vi "main2.vi"() -> ()   [LabVIEW 2012]
uses:
  Global1.vi
panel:
  out "String":string
  out "Lot":string
  in  "folder":string="QAMT01\\CRH3605"
  out "f":bool
  out "after substring":string
  out "before substring":string
  out "text":string
  out "error out":errorcluster
  in  "error in (no error)":errorcluster
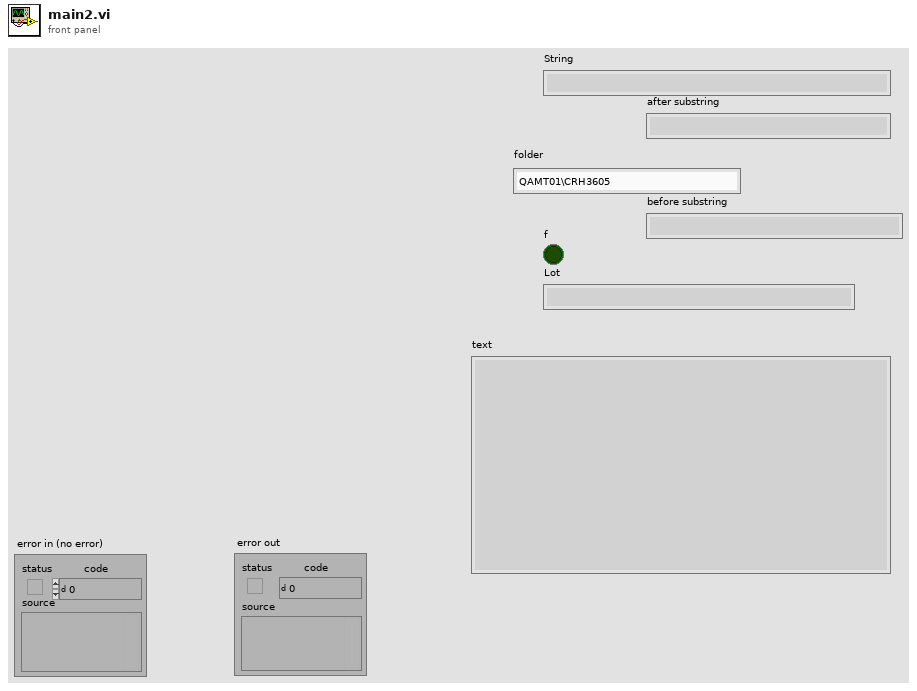
[diagram p1: front panel]
types:
  T1 = enum16{"open", "replace", "create", "open or create", "replace or create", "replace or create with confirmation"}
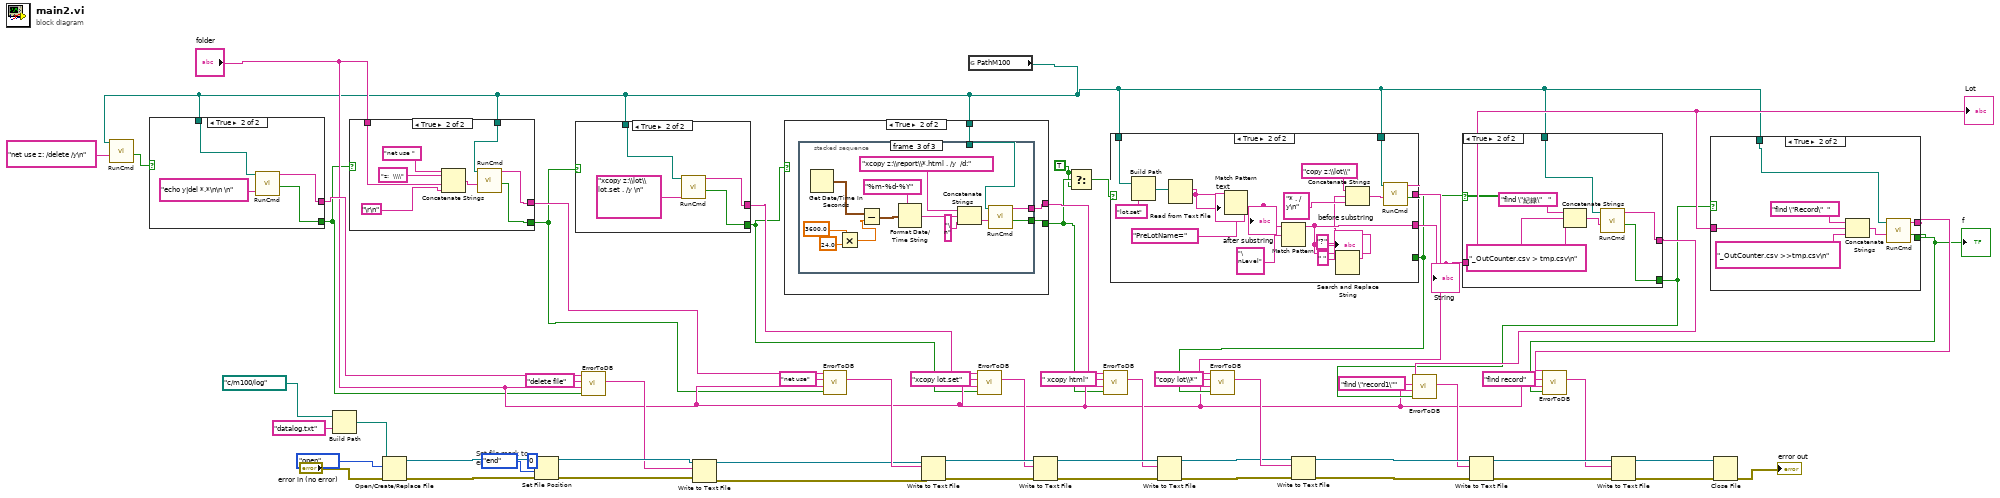
[diagram p0: block diagram]
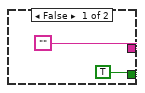
[diagram p2: hidden frame]
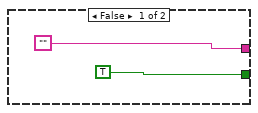
[diagram p3: hidden frame]
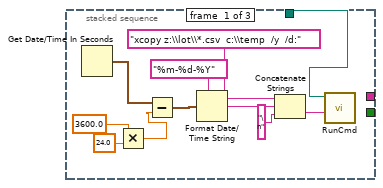
[diagram p4: hidden frame]
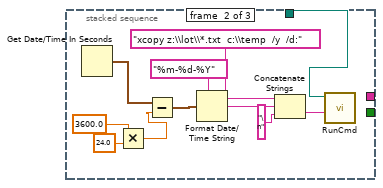
[diagram p5: hidden frame]
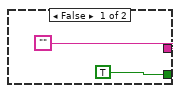
[diagram p6: hidden frame]
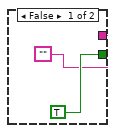
[diagram p7: hidden frame]
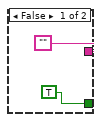
[diagram p8: hidden frame]
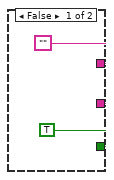
[diagram p9: hidden frame]
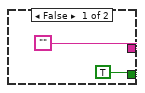
[diagram p10: hidden frame]
diagram:
  w6 = TRUE
  # "Set file mark to\nend of file"
  n1 = Build Path(base path=path "c:/m100/log", name or relative path="datalog.txt") -> (appended path=w53:path)
  n2 = Open/Create/Replace File(file path (use dialog)=w53, error in="error in (no error)", operation (0:open)=T1."open") -> (refnum out=w58:refnum<file>, error out=w57:errorcluster)  [unwired: 3 in, 1 out]
  n3 = Set File Position(offset (in bytes) (0)=i64 0, refnum=w58, from (0:start)=enum16{"start", "end", "current"}."end", error in=w57) -> (refnum out=w22:refnum<file>, error out=w21:errorcluster)
  n4 = global read "Global1.vi" "PathM100"() -> (w5:path)
  n5 = call "RunCmd.vi"("Cmd String"="net use z: /delete /y\n" ("string"), "working directory"=w5) -> ("OK"=w23:bool)  [unwired: 8 in, 1 out]
  n6 = case shown="True" w23 {
    tunnel: [TRUE w65] -> w3
    tunnel: ["" w64] -> w18
    tunnel: w5 -> [_ w67]
    frame False {
    }
    frame True {
      n7 = call "RunCmd.vi"("Cmd String"="echo y|del *.*\n\n \n" ("standard input"), "working directory"=w67) -> ("OK"=w65:bool, "Output"=w64:string)  [unwired: 8 in]
    }
  }
  n8 = case shown="True" w3 {
    tunnel: [TRUE w70] -> w4
    tunnel: ["" w71] -> w31
    tunnel: "folder" -> [_ w73]
    tunnel: w5 -> [_ w72]
    frame False {
    }
    frame True {
      n9 = Concatenate Strings("net use " ("string"), "z:  \\\\" ("string"), w73, "\r\n") -> (w77:string)
      n10 = call "RunCmd.vi"("Cmd String"=w77, "working directory"=w72) -> ("OK"=w70:bool, "Output"=w71:string)  [unwired: 8 in]
    }
  }
  n11 = case shown="True" w4 {
    tunnel: [TRUE w81] -> w2
    tunnel: ["" w80] -> w30
    tunnel: w5 -> [_ w83]
    frame False {
    }
    frame True {
      n12 = call "RunCmd.vi"("Cmd String"="xcopy z:\\lot\\lot.set . /y \n" ("standard input"), "working directory"=w83) -> ("OK"=w81:bool, "Output"=w80:string)  [unwired: 8 in]
    }
  }
  n13 = call "ErrorToDB.vi"("Error"=w3, "Folder"="folder", "Command"="delete file", "Error Message"=w18) -> ("LogData"=w17:string)  [unwired: 7 in]
  n14 = Write to Text File(file (use dialog)=w22, text=w17, error in=w21) -> (refnum out=w20:refnum<file>, error out=w19:errorcluster)  [unwired: 1 in, 1 out]
  n15 = case shown="True" w2 {
    tunnel: [TRUE w86] -> w8
    tunnel: ["" w87] -> w29
    tunnel: w5 -> [_ w88]
    frame False {
    }
    frame True {
      n16 = stacked-sequence {
        tunnel: w88 -> [w89 w100 w113]
        tunnel: [_ _ w112] -> w87
        tunnel: [_ _ w111] -> w86
        frame #0 {
          n17 = Get Date/Time In Seconds() -> (seconds since 1Jan1904=w90:timestamp)
          n18 = Multiply(x=3600.0, y=24.0) -> (x*y=w92:dbl)
          n19 = Subtract(x=w90, y=w92) -> (x-y=w93:timestamp)
          n20 = Format Date/Time String(time format string (%c)="%m-%d-%Y", seconds (now)=w93) -> (date/time string=w96:string)  [unwired: 1 in]
          n21 = Concatenate Strings("xcopy z:\\lot\\*.csv  c:\\temp  /y  /d:" ("string"), w96, "\n" ("string")) -> (w99:string)
          n22 = call "RunCmd.vi"("Cmd String"=w99, "working directory"=w89) -> ()  [unwired: 8 in, 2 out]
        }
        frame #1 {
          n23 = Get Date/Time In Seconds() -> (seconds since 1Jan1904=w101:timestamp)
          n24 = Multiply(x=3600.0, y=24.0) -> (x*y=w103:dbl)
          n25 = Subtract(x=w101, y=w103) -> (x-y=w104:timestamp)
          n26 = Format Date/Time String(time format string (%c)="%m-%d-%Y", seconds (now)=w104) -> (date/time string=w107:string)  [unwired: 1 in]
          n27 = Concatenate Strings("xcopy z:\\lot\\*.txt  c:\\temp  /y  /d:" ("string"), w107, "\n" ("string")) -> (w110:string)
          n28 = call "RunCmd.vi"("Cmd String"=w110, "working directory"=w100) -> ()  [unwired: 8 in, 2 out]
        }
        frame #2 {
          n29 = Get Date/Time In Seconds() -> (seconds since 1Jan1904=w114:timestamp)
          n30 = Multiply(x=3600.0, y=24.0) -> (x*y=w116:dbl)
          n31 = Subtract(x=w114, y=w116) -> (x-y=w117:timestamp)
          n32 = Format Date/Time String(time format string (%c)="%m-%d-%Y", seconds (now)=w117) -> (date/time string=w120:string)  [unwired: 1 in]
          n33 = Concatenate Strings("xcopy z:\\report\\*.html . /y  /d:" ("string"), w120, "\n" ("string")) -> (w123:string)
          n34 = call "RunCmd.vi"("Cmd String"=w123, "working directory"=w113) -> ("OK"=w111:bool, "Output"=w112:string)  [unwired: 8 in]
        }
      }
    }
  }
  n35 = call "ErrorToDB.vi"("Error"=w4, "Folder"="folder", "Command"="net use", "Error Message"=w31) -> ("LogData"=w43:string)  [unwired: 7 in]
  n36 = Write to Text File(file (use dialog)=w20, text=w43, error in=w19) -> (refnum out=w52:refnum<file>, error out=w51:errorcluster)  [unwired: 1 in, 1 out]
  n37 = call "ErrorToDB.vi"("Error"=w2, "Folder"="folder", "Command"="xcopy lot.set", "Error Message"=w30) -> ("LogData"=w42:string)  [unwired: 7 in]
  n38 = Write to Text File(file (use dialog)=w52, text=w42, error in=w51) -> (refnum out=w28:refnum<file>, error out=w27:errorcluster)  [unwired: 1 in, 1 out]
  n39 = Select(t=w6, s=w8, f=w6) -> (s? t:f=w7:bool)
  n40 = call "ErrorToDB.vi"("Error"=w8, "Folder"="folder", "Command"=" xcopy html", "Error Message"=w29) -> ("LogData"=w24:string)  [unwired: 7 in]
  n41 = case shown="True" w7 {
    tunnel: [TRUE w130] -> w38
    tunnel: [w124 w131] -> w39
    tunnel: w5 -> [_ w134]
    tunnel: [w124 w127] -> w44
    tunnel: w5 -> [_ w132]
    frame False {
      w124 = ""
    }
    frame True {
      n42 = Build Path(base path=w134, name or relative path="lot.set") -> (appended path=w142:path)
      n43 = Read from Text File(file (use dialog)=w142) -> (text=w139:string)  [unwired: 3 in, 3 out]
      "text" <- w139
      n44 = Match Pattern(string=w139, regular expression="PreLotName=") -> (after substring=w135:string)  [unwired: 1 in, 3 out]
      "after substring" <- w135
      n45 = Match Pattern(string=w135, regular expression="\nLevel") -> (before substring=w127:string)  [unwired: 1 in, 3 out]
      "before substring" <- w127
      n46 = Search and Replace String(input string=w127, search string=" ", replace string="?" ("replace string (\"\")")) -> (result string=w126:string)  [unwired: 5 in, 3 out]
      n47 = Concatenate Strings("copy z:\\lot\\" ("string"), w126, "* . /y\n" ("string")) -> (w133:string)
      n48 = call "RunCmd.vi"("Cmd String"=w133, "working directory"=w132) -> ("OK"=w130:bool, "Output"=w131:string)  [unwired: 8 in]
    }
  }
  "Lot" <- w44
  "String" <- w44
  n49 = Write to Text File(file (use dialog)=w28, text=w24, error in=w27) -> (refnum out=w26:refnum<file>, error out=w25:errorcluster)  [unwired: 1 in, 1 out]
  n50 = call "ErrorToDB.vi"("Error"=w38, "Folder"="folder", "Command"="copy lot\\*", "Error Message"=w39) -> ("LogData"=w40:string)  [unwired: 7 in]
  n51 = Write to Text File(file (use dialog)=w26, text=w40, error in=w25) -> (refnum out=w50:refnum<file>, error out=w49:errorcluster)  [unwired: 1 in, 1 out]
  n52 = case shown="True" w38 {
    tunnel: ["" w146] -> w36
    tunnel: w44 -> [_ w150]
    tunnel: w5 -> [_ w147]
    tunnel: [TRUE w145] -> w35
    frame False {
    }
    frame True {
      n53 = Concatenate Strings("find \"紀錄\"   " ("string"), w150, "_OutCounter.csv > tmp.csv\n" ("string")) -> (w148:string)
      n54 = call "RunCmd.vi"("Cmd String"=w148, "working directory"=w147) -> ("OK"=w145:bool, "Output"=w146:string)  [unwired: 8 in]
    }
  }
  n55 = call "ErrorToDB.vi"("Error"=w35, "Folder"="folder", "Command"="find \"record1\"", "Error Message"=w36) -> ("LogData"=w37:string)  [unwired: 7 in]
  n56 = Write to Text File(file (use dialog)=w50, text=w37, error in=w49) -> (refnum out=w48:refnum<file>, error out=w46:errorcluster)  [unwired: 1 in, 1 out]
  n57 = case shown="True" w35 {
    tunnel: w5 -> [_ w157]
    tunnel: w44 -> [_ w158]
    tunnel: ["" w154] -> w33
    tunnel: [TRUE w155] -> w32
    frame False {
    }
    frame True {
      n58 = Concatenate Strings("find \"Record\"  " ("string"), w158, "_OutCounter.csv >>tmp.csv\n" ("string")) -> (w156:string)
      n59 = call "RunCmd.vi"("Cmd String"=w156, "working directory"=w157) -> ("OK"=w155:bool, "Output"=w154:string)  [unwired: 8 in]
    }
  }
  "f" <- w32
  n60 = call "ErrorToDB.vi"("Error"=w32, "Folder"="folder", "Command"="find record", "Error Message"=w33) -> ("LogData"=w34:string)  [unwired: 7 in]
  n61 = Write to Text File(file (use dialog)=w48, text=w34, error in=w46) -> (refnum out=w47:refnum<file>, error out=w45:errorcluster)  [unwired: 1 in, 1 out]
  n62 = Close File(refnum=w47, error in=w45) -> (error out=→"error out":errorcluster)  [unwired: 1 out]
